vi "Log.Error.vi"(8 "error in":errorcluster, 9 "Append newline? (T)":bool=TRUE, 10 "Add to log file? (F)":bool, 11 "Message":string) -> (0 "error out":errorcluster)   [LabVIEW 2026, in "SystemMonitor Engine.lvlib" / "SystemMonitor Engine.lvclass"]
uses:
  SystemMonitor Engine.lvclass
  SystemMonitor Engine.lvclass/SystemMonitor Engine.ctl
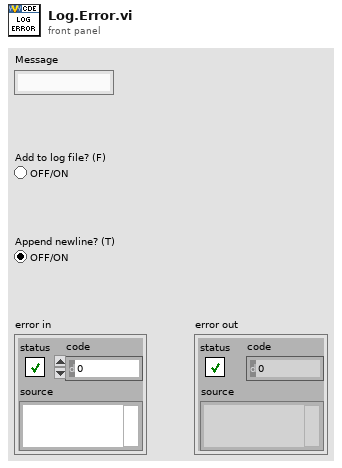
[diagram p1: front panel]
types:
  T1 = cluster{"Message":string, "Level":enum16{"Error", "Warning", "Info", "Debug"}, "Add to log file? (F)":bool, "Append newline? (T)":bool}
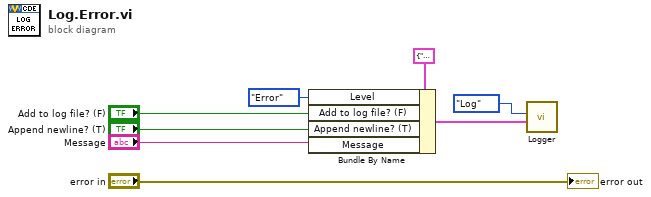
[diagram p0: block diagram]
diagram:
  n1 = Bundle By Name(cluster=T1 {"Message"="", "Level"=enum."Error", "Add to log file? (F)"=FALSE, "Append newline? (T)"=TRUE} ("Log"), "Level"=enum16{"Error", "Warning", "Info", "Debug"}."Error", "Add to log file? (F)"="Add to log file? (F)", "Append newline? (T)"="Append newline? (T)", "Message"="Message") -> (w3:T1)
  n2 = call "Logger.vi"("Log"=w3, "State"=enum16{"Initialize", "Log"}."Log") -> ()  [unwired: 8 in, 2 out]
  "error out" <- "error in"
